vi "Find highest intensity filter position.vi"(8 "error in":errorcluster, 10 "No of points":i32=2, 11 "VISA resource name out":refnum<visa-resource-name>) -> (0 "error out":errorcluster, 3 "Angle to no filter (deg.)":sgl)   [LabVIEW 2011]
uses:
  <instrlib>/keithley_24xx/Keithley 24XX/Public/Data/Read (Multiple Points).vi
  <instrlib>/keithley_24xx/Keithley 24XX/Keithley 24XX.lvlib
panel:
  out "Average time step (ms)":sgl
  out "Measurement times (s)":sgl[](array[numeric])
  out "J-t":sgl[][](array[numeric]) format="%#_11g"
  out "J-t":cluster{sgl[], sgl[]}(graph)
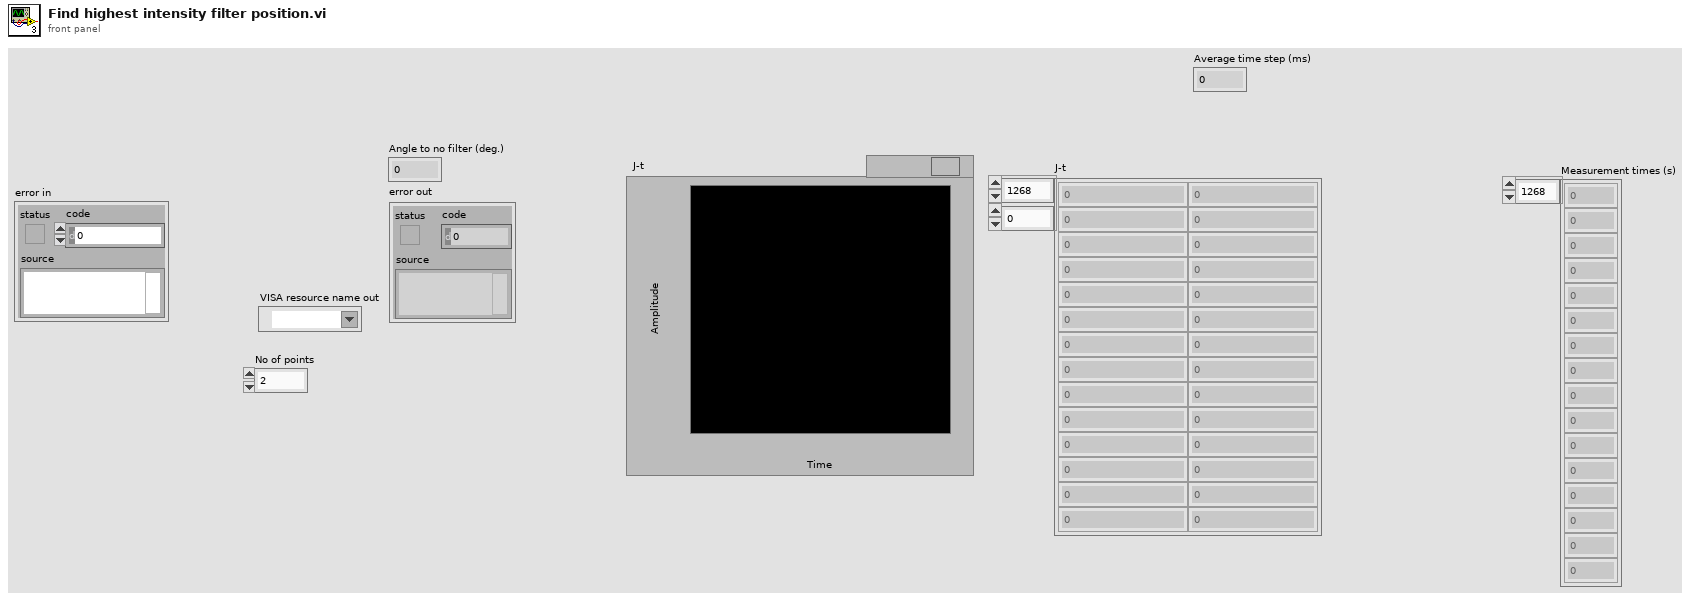
[diagram p1: front panel]
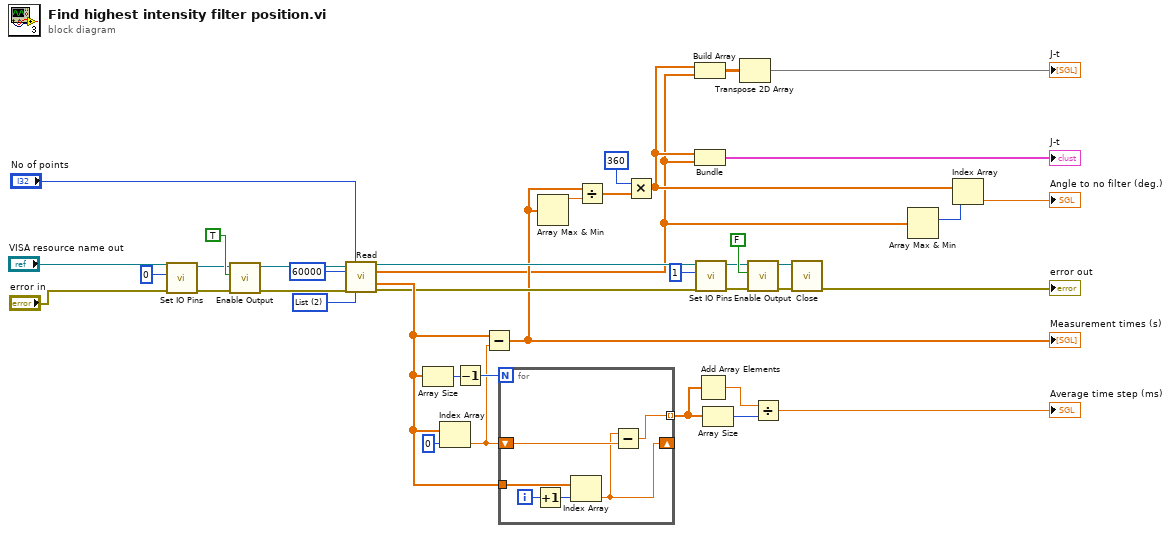
[diagram p0: block diagram]
diagram:
  w16 = u16 2 items=["Fixed", "Sweep", "List"] ("Output Mode (0: Fixed)")
  n1 = call <instrlib>:"Set IO Pins.vi"("error in (no error)"="error in", "Output Pattern (0)"=0, "VISA resource name"="VISA resource name out") -> ("error out"=w3:errorcluster, "VISA resource name out"=w5:refnum<visa-resource-name>)  [unwired: 7 in]
  n2 = call <instrlib>:"Enable Output.vi"("error in (no error)"=w3, "Enable Output (T: Enable)"=TRUE ("Output (Off)"), "VISA resource name"=w5) -> ("error out"=w8:errorcluster, "VISA resource name out"=w9:refnum<visa-resource-name>)  [unwired: 7 in]
  n3 = call-poly <instrlib>:"Read.vi"("VISA resource name"=w9, "Sample Count (1)"="No of points", "Timeout (10000 ms)"=60000, "error in (no error)"=w8, "Output Mode (0: Fixed)"=w16) -> ("VISA resource name out"=w14:refnum<visa-resource-name>, "Current"=w1:sgl[], "Timestamp"=w13:sgl[], "error out"=w12:errorcluster)  [unwired: 4 in, 3 out]
  n4 = Array Size(array=w13) -> (size(s)=w24:i32)
  n5 = Index Array(array=w13, index=0) -> (element=w23:sgl)
  n6 = Decrement(x=w24) -> (x-1=w25:i32)
  n7 = Subtract(x=w13, y=w23) -> (x-y=w2:sgl[])
  "Measurement times (s)" <- w2
  n8 = for {
    N: w25 -> [_]
    tunnel: w13 -> [w44]
    shift-right: [w42] -> _
    shift-left: w23 -> [w43]
    tunnel: [w41] -> w33 mode=indexing
    i -> [w46]
    n9 = Increment(x=w46) -> (x+1=w45:i32)
    n10 = Index Array(array=w44, index=w45) -> (element=w42:sgl)
    n11 = Subtract(x=w42, y=w43) -> (x-y=w41:sgl)
  }
  n12 = Array Max & Min(array=w2) -> (max value=w22:sgl)  [unwired: 3 out]
  n13 = Divide(x=w2, y=w22) -> (x/y=w21:sgl[])
  n14 = Multiply(x=360, y=w21) -> (x*y=w19:sgl[])
  n15 = Build Array(w19, w1) -> (w27:sgl[][])
  n16 = Bundle(w19, "Current"=w1) -> (→"J-t":cluster{sgl[], "Current":sgl[]})  [unwired: 1 in]
  n17 = call <instrlib>:"Set IO Pins.vi"("error in (no error)"=w12, "Output Pattern (0)"=1, "VISA resource name"=w14) -> ("error out"=w35:errorcluster, "VISA resource name out"=w37:refnum<visa-resource-name>)  [unwired: 7 in]
  n18 = Add Array Elements(numeric array=w33) -> (sum=w31:sgl)
  n19 = Array Size(array=w33) -> (size(s)=w32:i32)
  n20 = Transpose 2D Array(2D array=w27) -> (transposed array=→"J-t":sgl[][])
  n21 = call <instrlib>:"Enable Output.vi"("error in (no error)"=w35, "Enable Output (T: Enable)"=FALSE ("Output (Off)"), "VISA resource name"=w37) -> ("error out"=w39:errorcluster, "VISA resource name out"=w40:refnum<visa-resource-name>)  [unwired: 7 in]
  n22 = Divide(x=w31, y=w32) -> (x/y=→"Average time step (ms)":sgl)
  n23 = call <instrlib>:"Close.vi"("error in (no error)"=w39, "VISA resource name"=w40) -> ("error out"=→"error out":errorcluster)  [unwired: 9 in]
  n24 = Array Max & Min(array=w1) -> (max index (indices)=w18:i32)  [unwired: 3 out]
  n25 = Index Array(array=w19, index=w18) -> (element=→"Angle to no filter (deg.)":sgl)
